vi "Property Node_Unwired Terminals.vi"(8 "error in":errorcluster, 11 "Property Node Ref":refnum<vi>) -> (0 "error out":errorcluster, 1 "Unwired Indices For Removal":i32[](array[numeric]), 2 "Unwired Indices":i32[](array[numeric]), 3 "Property Items[]":refnum<vi>[](array[refnum]))   [LabVIEW 2023]
doc: "Returns list of unwired terminals, and a separate list of those the can be removed. The latter will be different if all terminals are unwired, because you cannot remove *all* unwired terminals from the node."
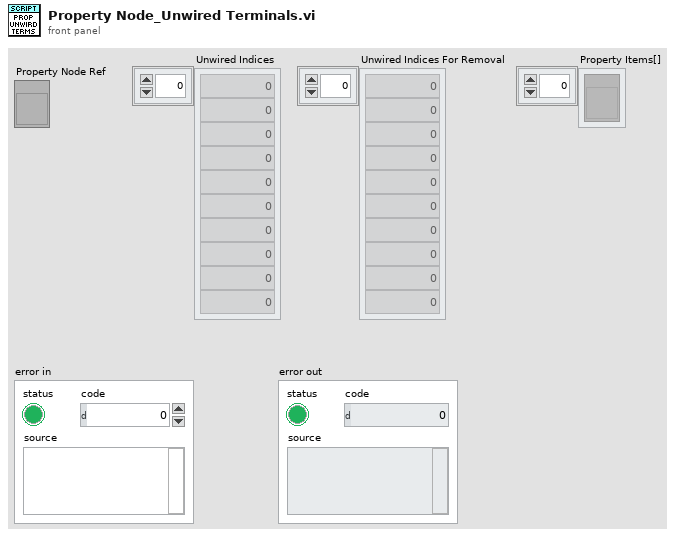
[diagram p1: front panel]
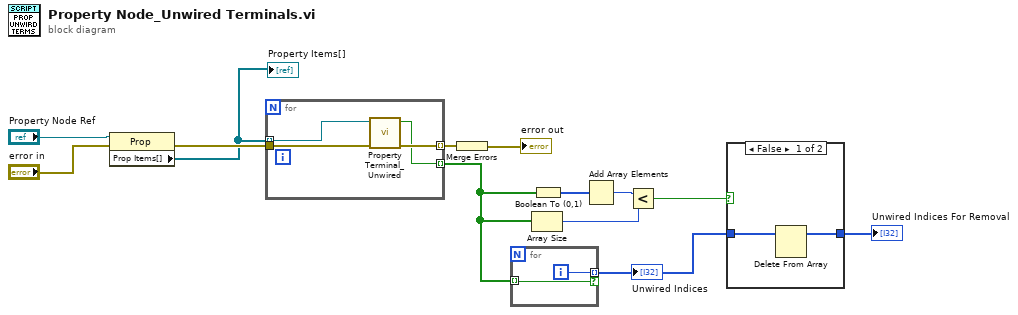
[diagram p0: block diagram]
diagram:
  n1 = property class="Prop"(reference="Property Node Ref", error in="error in") -> (error out=w7:errorcluster, "Prop Items[]"=w6:refnum<vi>[])  [unwired: 1 out]
  "Property Items[]" <- w6
  n2 = for {
    tunnel: w6 -> [w17] mode=indexing
    tunnel: [w14] -> w5 mode=indexing
    tunnel: w7 -> [w16]
    tunnel: [w15] -> w4 mode=indexing
    n3 = call "Property Terminal_Unwired.vi"("error in"=w16, "PropertyItem in"=w17) -> ("error out"=w15:errorcluster, "Unwired"=w14:bool)  [unwired: 7 in, 1 out]
  }
  n4 = Merge Errors(w4) -> (→"error out":errorcluster)
  n5 = for {
    tunnel: w5 -> [w19] mode=indexing
    tunnel: [w18] -> w12 mode=indexing if=w19
    i -> [w18]
  }
  "Unwired Indices" <- w12
  n6 = Array Size(array=w5) -> (size(s)=w2:i32)
  n7 = Boolean To (0,1)(Boolean=w5) -> (0, 1=w13:i16[])
  n8 = Add Array Elements(numeric array=w13) -> (sum=w3:i16)
  n9 = Less?(x=w3, y=w2) -> (x < y?=w1:bool)
  n10 = case shown="False" w1 {
    tunnel: w12 -> [w21 w22]
    tunnel: [w20 w22] -> w11
    frame False {
      n11 = Delete From Array(array=w21) -> (array with subset deleted=w20:i32[])  [unwired: 2 in, 1 out]
    }
    frame True {
    }
  }
  "Unwired Indices For Removal" <- w11
